vi "WriteToCSV.vi"(0 "Pages":refnum<vi>[](array[refnum]), 1 "file path (dialog if empty)":path) -> (2 "output array for NT":string[](array[string]))   [LabVIEW 2019]
uses:
  <vilib>/Utility/file.llb/Write Delimited Spreadsheet (string).vi
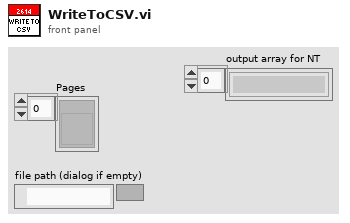
[diagram p1: front panel]
types:
  T1 = enum16{"open", "replace", "create", "open or create", "replace or create", "replace or create with confirmation"}
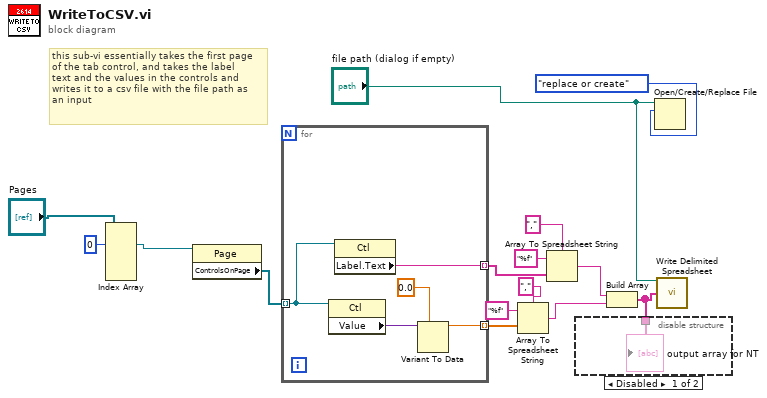
[diagram p0: block diagram]
diagram:
  # "this sub-vi essentially takes the first page\nof the tab control, and takes the label\ntext and the values in the controls and \nwrites it to a csv file with the file path as\nan input"
  n1 = Index Array(array="Pages", index #1=0 ("index")) -> (element #1=w14:refnum<vi>)  [unwired: 4 in, 4 out]
  n2 = property class="Page"(reference=w14) -> ("ControlsOnPage"=w6:refnum<vi>[])  [unwired: 1 in, 2 out]
  n3 = for {
    tunnel: w6 -> [w19] mode=indexing
    tunnel: [w20] -> w5 mode=indexing
    tunnel: [w17] -> w1 mode=indexing
    n4 = property class="Ctl"(reference=w19) -> ("Value"=w18:variant)  [unwired: 1 in, 2 out]
    n5 = property class="Ctl"(reference=w19) -> ("Label.Text"=w20:string)  [unwired: 1 in, 2 out]
    n6 = Variant To Data(type=0.0, Variant=w18) -> (data=w17:dbl)  [unwired: 1 in, 1 out]
  }
  n7 = Array To Spreadsheet String(delimiter (Tab)=",", array=w1, 3:"%f" ("format string")) -> (spreadsheet string=w3:string)
  n8 = Array To Spreadsheet String(delimiter (Tab)=",", array=w5, 3:"%f" ("format string")) -> (spreadsheet string=w4:string)
  n9 = Build Array(w4, w3) -> (w2:string[])
  n10 = disable-structure shown="Disabled" {
    disable-tunnel: w2 -> [w21 _]
    frame Disabled {
      "output array for NT" <- w21
    }
    frame Enabled {
    }
  }
  n11 = Open/Create/Replace File(file path (use dialog)="file path (dialog if empty)", operation (0:open)=T1."replace or create") -> ()  [unwired: 4 in, 3 out]
  n12 = call-poly <vilib>:"Write Delimited Spreadsheet.vi"("file path (dialog if empty)"="file path (dialog if empty)", "1D data"=w2) -> ()  [unwired: 12 in, 2 out]
